vi "Read Waveform (Single).vi"(8 "error in (no error)":errorcluster, 9 "Maximum Time (10000 ms)":u32=10000, 10 "Channel (1: Channel 1)":u16(ring)=1 items=["Channel 1"=1, "Channel 2"=2], 11 "VISA resource name":refnum<visa-resource-name>) -> (0 "error out":errorcluster, 2 "Waveform Data":waveform(dbl)(graph), 3 "VISA resource name out":refnum<visa-resource-name>)   [LabVIEW 2013, in "Template - Scope.lvlib"]
doc: "Initiates an acquisition on all channels that you enabled with the Configure Channel VI. The VI waits for the acquisition to complete and returns the waveform for the <B>Source Channel</B> you specified. If the oscilloscope did not complete the acquisition within the time period you specify with the <B>Timeout</B> control, the VI returns a timeout error. A common cause for a timeout error is the acquisition was not triggered. For example, the trigger level is out of range of the waveform.\n\nCall the Fetch Waveform VI to obtain the waveforms for each of the remaining enabled <B>Source Channels</B> without initiating another acquisition.\n\n<B>Note:</B> If your instrument does not support auto compensation for probe attenuation, you may need to adjust the scaling of the Waveform Data accordingly. This is handled automatically in the <B>Configure Channel</B> VI or can be done manually by multiplying the <B>Waveform Data</B> by the probe attenuation."
uses:
  <instrlib>/_Template - Scope/Template - Scope.lvlib
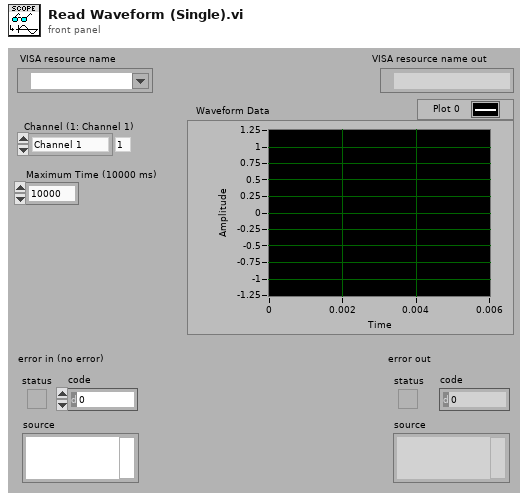
[diagram p1: front panel]
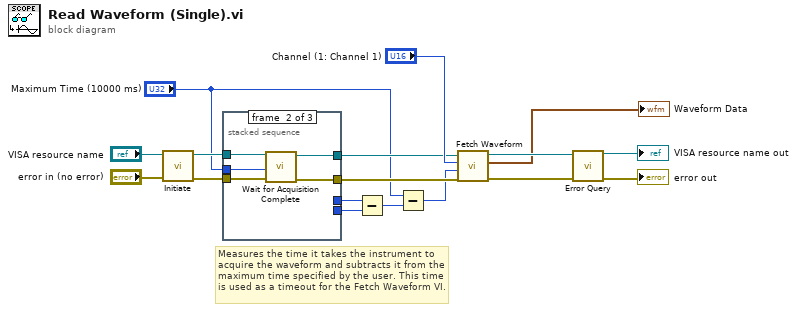
[diagram p0: block diagram]
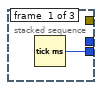
[diagram p2: hidden frame]
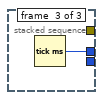
[diagram p3: hidden frame]
diagram:
  # "Measures the time it takes the instrument to acquire the waveform and subtracts it from the maximum time specified by the user. This time is used as a timeout for the Fetch Waveform VI."
  n1 = call <instrlib>:"Initiate.vi"("error in (no error)"="error in (no error)", "VISA resource name"="VISA resource name") -> ("error out"=w7:errorcluster, "VISA resource name out"=w9:refnum<visa-resource-name>)  [unwired: 8 in]
  n2 = stacked-sequence {
    tunnel: w9 -> [_ w23 _]
    tunnel: [_ w22 _] -> w8
    tunnel: w7 -> [_ w21 _]
    tunnel: [_ w20 _] -> w6
    tunnel: "Maximum Time (10000 ms)" -> [_ w19 _]
    tunnel: [w18 _ _] -> w2
    tunnel: [_ _ w24] -> w1
    frame #0 {
      n3 = Tick Count (ms)() -> (millisecond timer value=w18:u32)
    }
    frame #1 {
      n4 = call <instrlib>:"Wait for Acquisition Complete.vi"("error in (no error)"=w21, "Maximum Time (10000 ms)"=w19, "VISA resource name"=w23) -> ("error out"=w20:errorcluster, "VISA resource name out"=w22:refnum<visa-resource-name>)  [unwired: 7 in]
    }
    frame #2 {
      n5 = Tick Count (ms)() -> (millisecond timer value=w24:u32)
    }
  }
  n6 = Subtract(x=w1, y=w2) -> (x-y=w5:u32)
  n7 = Subtract(x="Maximum Time (10000 ms)", y=w5) -> (x-y=w3:u32)
  n8 = call <instrlib>:"Fetch Waveform.vi"("error in (no error)"=w6, "Timeout (10000 ms)"=w3, "Channel (1: Channel 1)"="Channel (1: Channel 1)", "VISA resource name"=w8) -> ("error out"=w11:errorcluster, "Waveform Data"=→"Waveform Data":waveform(dbl), "VISA resource name out"=w12:refnum<visa-resource-name>)  [unwired: 5 in]
  n9 = call <instrlib>:"Error Query.vi"("error in (no error)"=w11, "VISA resource name"=w12) -> ("error out"=→"error out":errorcluster, "VISA resource name out"=→"VISA resource name out":refnum<visa-resource-name>)  [unwired: 6 in, 2 out]
